vi "Configure Feed Forward Equalization Tap Optimization.vi"(6 "Eye Width (0.333)":dbl=0.333, 8 "error in (no error)":errorcluster, 9 "Custom Pattern (\"\")":string, 10 "Pattern (1: 2^5-1)":i32(ring)=1 items=["2^5-1"=1, "2^6-1"=2, "2^7-1"=3, "2^8-1"=4, "2^9-1"=5, "2^10-1"=6, "Custom Pattern"=0], 11 "VISA resource name":refnum<visa-resource-name>) -> (0 "error out":errorcluster, 3 "VISA resource name out":refnum<visa-resource-name>)   [LabVIEW 2020, in "Agilent 90000 Series.lvlib"]
doc: "Configures the optimization parameters for Feed-Forward Equalization."
uses:
  Agilent 90000 Series.lvlib
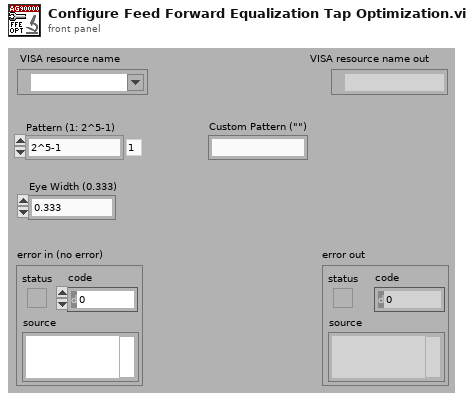
[diagram p1: front panel]
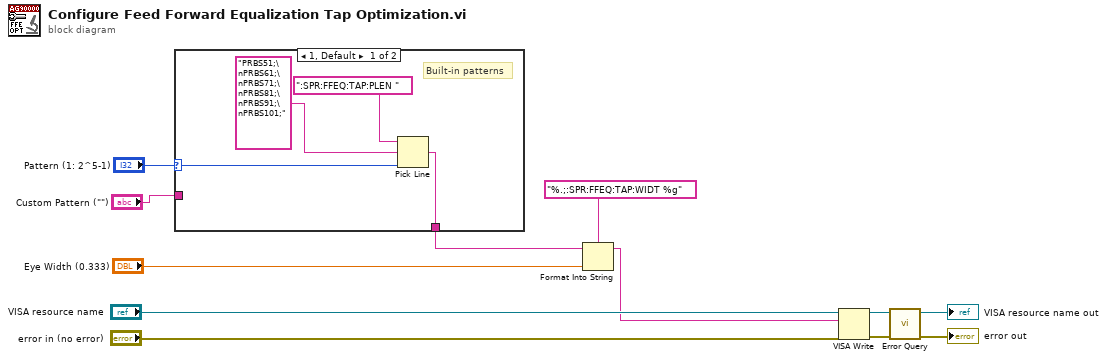
[diagram p0: block diagram]
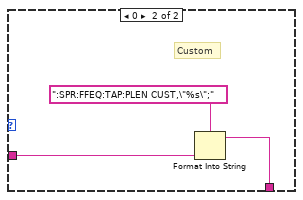
[diagram p2: hidden frame]
diagram:
  n1 = case shown="1, Default" "Pattern (1: 2^5-1)" {
    selector: "Pattern (1: 2^5-1)" -> [w16 _]
    tunnel: "Custom Pattern (\"\")" -> [_ w18]
    tunnel: [w13 w17] -> w3
    frame 1, Default {
      # "Built-in patterns"
      n2 = Pick Line(string ("")=":SPR:FFEQ:TAP:PLEN ", multi-line string="PRBS51;\nPRBS61;\nPRBS71;\nPRBS81;\nPRBS91;\nPRBS101;", line index=w16) -> (output string=w13:string)
    }
    frame 0 {
      # "Custom"
      n3 = Format Into String(format string=":SPR:FFEQ:TAP:PLEN CUST,\"%s\";", w18) -> (resulting string=w17:string)  [unwired: 2 in, 1 out]
    }
  }
  n4 = Format Into String(format string="%.;:SPR:FFEQ:TAP:WIDT %g", initial string=w3, "Eye Width (0.333)") -> (resulting string=w1:string)  [unwired: 1 in, 1 out]
  n5 = VISA Write(VISA resource name="VISA resource name", write buffer=w1, error in (no error)="error in (no error)") -> (VISA resource name out=w10:refnum<visa-resource-name>, error out=w9:errorcluster)  [unwired: 1 out]
  n6 = call "Error Query.vi"("error in (no error)"=w9, "VISA resource name"=w10) -> ("error out"=→"error out":errorcluster, "VISA resource name out"=→"VISA resource name out":refnum<visa-resource-name>)  [unwired: 8 out]
